vi "Init.vi"(8 "error in (no error)":errorcluster, 9 "size(KB)":u32, 10 "Name":string, 11 "LogRotate in":refnum<class "LogRotate.lvclass">) -> (0 "error out":errorcluster, 3 "LogRotate out":refnum<class "LogRotate.lvclass">)   [LabVIEW 2019, in "Error_Manager.lvlib" / "LogRotate.lvclass"]
uses:
  LogRotate.lvclass
  LogData.ctl
  LogRotate.lvclass/LogRotate.ctl
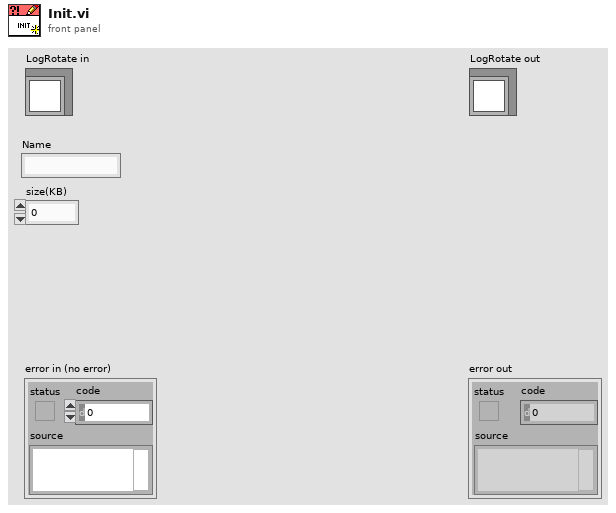
[diagram p1: front panel]
types:
  T1 = typedef "Error_Manager.lvlib/LogRotate.lvclass/LogData.ctl" = cluster{"error constant":errorcluster, "replacements":string[], "Time Stamp":timestamp}
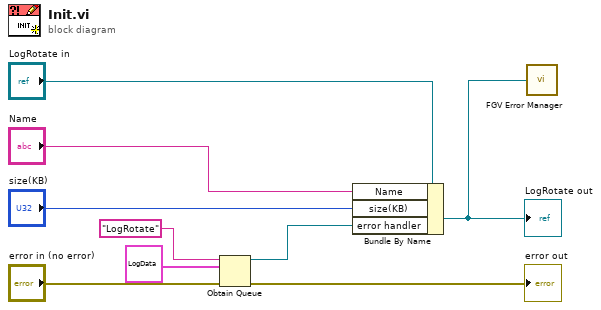
[diagram p0: block diagram]
diagram:
  n1 = Obtain Queue(name (unnamed)="LogRotate", element data type=T1 {"error constant"={"status"=FALSE, "code"=0, "source"=""}, "replacements"=[], "Time Stamp"=timestamp(0 s since 1904-01-01)} ("LogData"), error in (no error)="error in (no error)") -> (queue out=w4:refnum<queue>, error out=→"error out":errorcluster)  [unwired: 2 in, 1 out]
  n2 = Bundle By Name(cluster="LogRotate in", "Name"="Name", "size(KB)"="size(KB)", "error handler"=w4) -> (w2:refnum<class "LogRotate.lvclass">)
  "LogRotate out" <- w2
  n3 = call "FGV Error Manager.vi"("error_manager in"=w2) -> ()  [unwired: 1 out]
